vi "arduino_2_0.vi"() -> ()   [LabVIEW 2015]
uses:
  <vilib>/LabVIEW Interface for Arduino/LabVIEW Interface for Arduino.lvlib
panel:
  out "Waveform Chart":dbl(graph)
  in  "stop":bool
  out "Potentiometer":dbl(knob) scale=0.0..5.0
  in  "Analog Input Pin (0)":u8
  in  "VISA resource":refnum<visa-resource-name>
  # "Connect potentiometer arduino pin A0 when you rotate potentiometer in labview show"
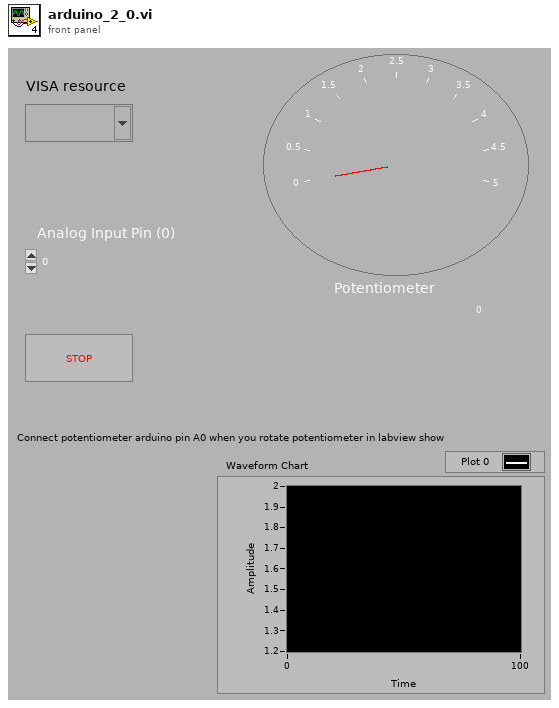
[diagram p1: front panel]
types:
  T1 = typedef "LabVIEW Interface for Arduino.lvlib/Arduino Resource.ctl" = cluster{"VISA resource":refnum<visa-resource-name>, "Board Type":T2, "Connection Type":enum8{"USB / Serial"}, "Bytes Per Packet (15)":u8}
  T2 = typedef "LabVIEW Interface for Arduino.lvlib/Board Type.ctl" = enum16{"Uno", "Dimuelanove w/Atmega 328", "Mega 2560"}
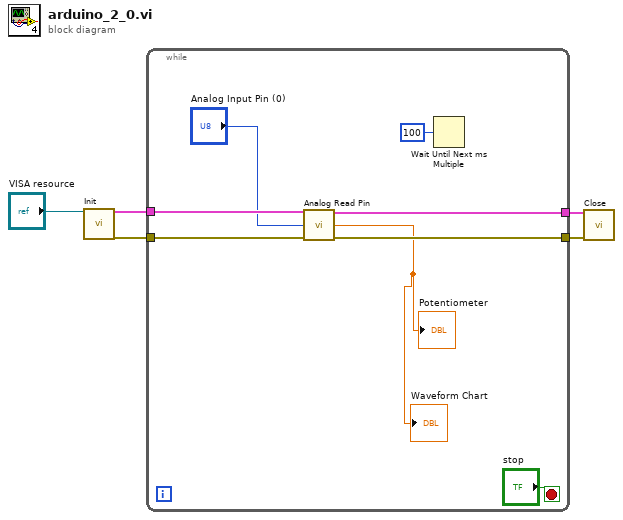
[diagram p0: block diagram]
diagram:
  n1 = call <vilib>:"Init.vi"("VISA resource"="VISA resource") -> ("Arduino Resource"=w5:T1, "error out"=w3:errorcluster)  [unwired: 17 in]
  n2 = while {
    tunnel: w5 -> [w13]
    tunnel: [w12] -> w4
    tunnel: w3 -> [w11]
    tunnel: [w10] -> w2
    stop <- "stop" stop-if-true
    n3 = call <vilib>:"Analog Read Pin.vi"("Arduino Resource"=w13, "Analog Input Pin (0)"="Analog Input Pin (0)", "error in"=w11) -> ("Arduino Resource"=w12:T1, "Voltage"=→"Potentiometer" →"Waveform Chart":dbl, "error out"=w10:errorcluster)  [unwired: 10 in]
    n4 = Wait Until Next ms Multiple(millisecond multiple=u32 100) -> ()  [unwired: 1 out]
  }
  n5 = call <vilib>:"Close.vi"("Arduino Resource"=w4, "error in"=w2) -> ()  [unwired: 13 in, 1 out]
